vi "Configure Marker State.vi"(7 "Marker On":bool, 8 "error in (no error)":errorcluster, 10 "Marker Number":u8=1, 11 "VNA-CMT S2 S4 in":refnum<class "VNA-CMT S2 S4.lvclass">) -> (0 "error out":errorcluster, 3 "VNA-CMT S2 S4 out":refnum<class "VNA-CMT S2 S4.lvclass">)   [LabVIEW 2020, in "VNA-CMT S2 S4.lvclass"]
doc: "Configure the marker state.\nThe marker is on the active trace."
uses:
  VNA-CMT S2 S4.lvclass
  C:/Sandbox/RF Bench/Source Code/WiSpry Test Framework/Instruments/Instrument.lvclass
  Instrument.lvclass/Instrument.ctl
  Instrument.lvclass
  <instrlib>/CMT S2 and S4 VNA/CMT S2 and S4 VNA.lvlib
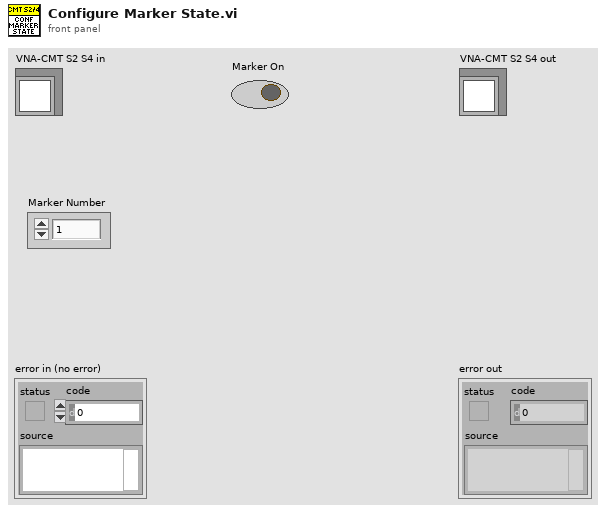
[diagram p1: front panel]
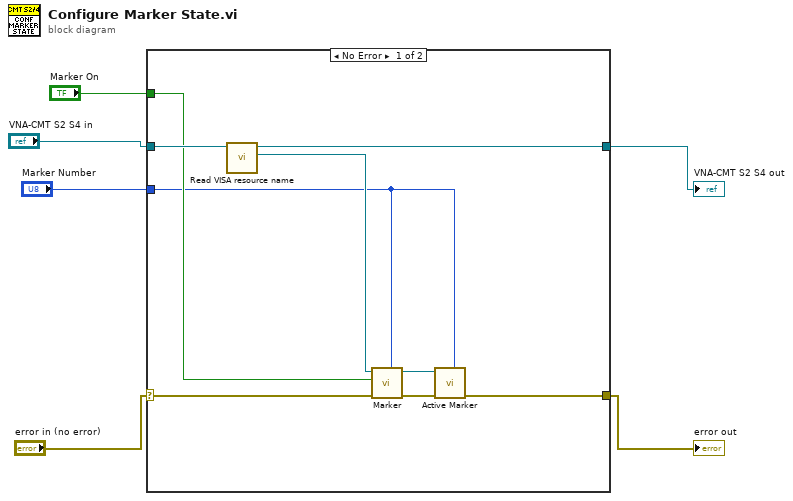
[diagram p0: block diagram]
diagram:
  n1 = case shown="No Error" "error in (no error)" {
    selector: "error in (no error)" -> [w10 w16]
    tunnel: "VNA-CMT S2 S4 in" -> [w15 w17]
    tunnel: [w14 w17] -> w4
    tunnel: [w9 w16] -> w5
    tunnel: "Marker On" -> [w8 _]
    tunnel: "Marker Number" -> [w7 _]
    frame No Error {
      n2 = call "Read VISA resource name.vi"("Instrument in"=w15) -> ("VISA resource name"=w11:refnum<visa-resource-name>, "Instrument out"=w14:refnum<class "VNA-CMT S2 S4.lvclass">)  [unwired: 9 in]
      n3 = call <instrlib>:"Marker.vi"("Marker (1)"=w7, "error in (no error)"=w10, "Marker State (F: Disabled)"=w8, "VISA resource name"=w11) -> ("error out"=w12:errorcluster, "VISA resource name out"=w13:refnum<visa-resource-name>)  [unwired: 6 in]
      n4 = call <instrlib>:"Active Marker.vi"("Marker (1)"=w7, "error in (no error)"=w12, "VISA resource name"=w13) -> ("error out"=w9:errorcluster)  [unwired: 7 in, 1 out]
    }
    frame Error {
    }
  }
  "error out" <- w5
  "VNA-CMT S2 S4 out" <- w4
